vi "Test State Name Parser.vi"   [LabVIEW 2013]
uses:
  <vilib>/addons/_JKI Toolkits/Caraya/classes/Assert/Assert.lvclass
  <vilib>/addons/_JKI Toolkits/Caraya/classes/Test/Test.lvclass
  source/JKI SM/JKI SM.lvclass
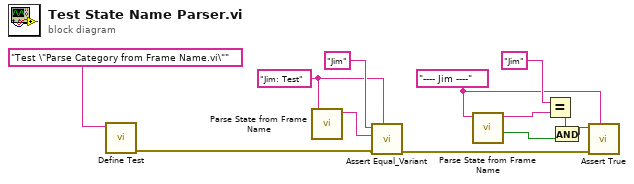
[diagram p0: block diagram]
diagram:
  w3 = "---- Jim ----" ("Frame Name")
  w5 = "Jim: Test" ("Frame Name")
  n1 = call <vilib>:"Define Test.vi"("Label (VI Title)"="Test \"Parse Category from Frame Name.vi\"") -> ("error out"=w10:errorcluster)  [unwired: 10 in]
  n2 = call "Parse State from Frame Name.vi"("Frame Name"=w5) -> ("Category Name"=w4:string)  [unwired: 7 in, 3 out]
  n3 = call <vilib>:"Assert Equal_Variant.vi"("Label"=w5, "error in (no error)"=w10, "Y"=w4, "X"="Jim" ("Frame Name")) -> ("error out"=w9:errorcluster)  [unwired: 7 in]
  n4 = call "Parse State from Frame Name.vi"("Frame Name"=w3) -> ("is a Category Frame?"=w1:bool, "Category Name"=w2:string)  [unwired: 7 in, 2 out]
  n5 = Equal?(x="Jim" ("Frame Name"), y=w2) -> (x = y?=w7:bool)
  n6 = And(x=w7, y=w1) -> (x .and. y?=w6:bool)
  n7 = call <vilib>:"Assert True.vi"("Label"=w3, "error in (no error)"=w9, "True?"=w6) -> ()  [unwired: 8 in, 1 out]
